vi "Read DMAs.vi"(8 "Number of Elements":u32, 11 "FPGA VI Reference In":refnum<k20>) -> (0 "Next Amp":dbl[](array[numeric]), 1 "Prev Amp":dbl[](array[numeric]), 2 "Max Amp":dbl[](array[numeric]), 3 "Max bin":dbl[](array[numeric]), 4 "Elements Remaining in Max bin DMA":u32, 6 "error out":errorcluster)   [LabVIEW 2014]
doc: "This subVI reads the DMA in parallel"
uses:
  <vilib>/Utility/error.llb/Error Cluster From Error Code.vi
  <vilib>/rvi/errors/niLvFpgaAdjustHostInterfaceError.vi
  <vilib>/rvi/interface/nirviMethod/nirviMethod.xnode
  <vilib>/FPGAPlugInAG/Dynamic/niLvFpga_ReadFifo_Dynamic.vi
  <vilib>/rvi/errors/niLvFpgaMergeErrorWithErrorCode.vi
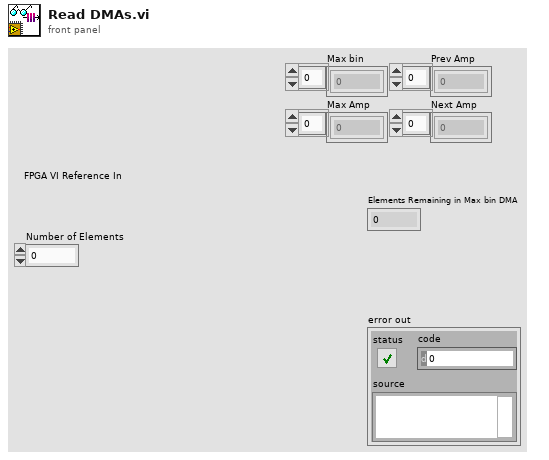
[diagram p1: front panel]
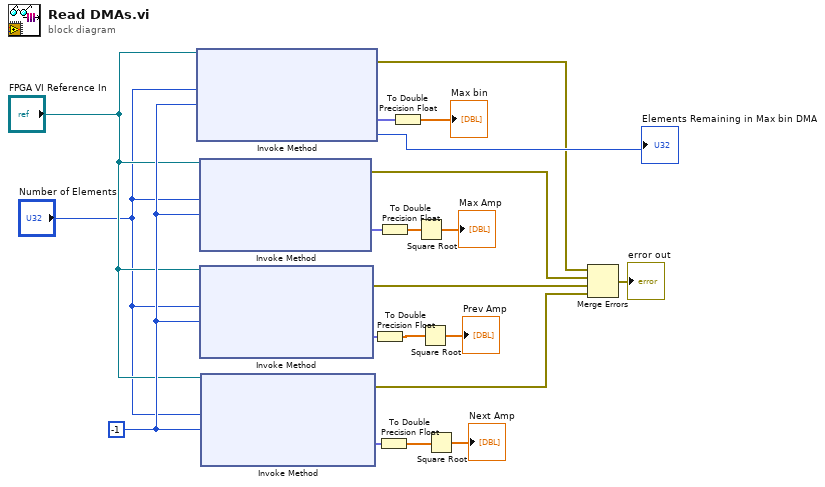
[diagram p0: block diagram]
diagram:
  w14 = -1 ("Timeout (ms)")
  n1 = xnode "Invoke Method"("FPGA VI Reference In"="FPGA VI Reference In", "Number of Elements"="Number of Elements", "Timeout (ms)"=w14) -> ("error out"=w2:errorcluster, "Data"=w13:fxp<+/-,12,12>[], "Elements Remaining"=→"Elements Remaining in Max bin DMA":u32)  [unwired: 1 in, 1 out]
  n2 = xnode "Invoke Method"("FPGA VI Reference In"="FPGA VI Reference In", "Number of Elements"="Number of Elements", "Timeout (ms)"=w14) -> ("error out"=w3:errorcluster, "Data"=w20:fxp<+,44,44>[])  [unwired: 1 in, 2 out]
  n3 = xnode "Invoke Method"("FPGA VI Reference In"="FPGA VI Reference In", "Number of Elements"="Number of Elements", "Timeout (ms)"=w14) -> ("error out"=w4:errorcluster, "Data"=w18:fxp<+,44,44>[])  [unwired: 1 in, 2 out]
  n4 = xnode "Invoke Method"("FPGA VI Reference In"="FPGA VI Reference In", "Number of Elements"="Number of Elements", "Timeout (ms)"=w14) -> ("error out"=w5:errorcluster, "Data"=w16:fxp<+,44,44>[])  [unwired: 1 in, 2 out]
  n5 = To Double Precision Float(number=w18) -> (double precision float=w17:dbl[])
  n6 = To Double Precision Float(number=w16) -> (double precision float=w15:dbl[])
  n7 = To Double Precision Float(number=w20) -> (double precision float=w19:dbl[])
  n8 = To Double Precision Float(number=w13) -> (double precision float=→"Max bin":dbl[])
  n9 = Square Root(x=w19) -> (sqrt(x)=→"Max Amp":dbl[])
  n10 = Square Root(x=w17) -> (sqrt(x)=→"Prev Amp":dbl[])
  n11 = Square Root(x=w15) -> (sqrt(x)=→"Next Amp":dbl[])
  n12 = Merge Errors(w2, w3, w4, w5) -> (→"error out":errorcluster)
